vi "Test Snake Created Outside World.vi"(8 "error in (no error)":errorcluster, 11 "Test Case In":refnum<class "World Test.lvclass">) -> (0 "error out":errorcluster, 3 "Test Case Out":refnum<class "World Test.lvclass">)   [LabVIEW 2020, in "World Test.lvclass"]
uses:
  World Test.lvclass
  World Test.lvclass/World Test.ctl
  source/World/World.lvclass
  source/Particle/Position.ctl
  source/Particle.lvclass
  source/Snake/Snake.lvclass
  <vilib>/Astemes/LUnit/Test Case.lvclass
  C:/Program Files (x86)/National Instruments/LabVIEW 2020/vi.lib/Astemes/LUnit/Test Case.lvclass
  C:/git/astemes-snake-game/tests/World Test/World Test.lvclass
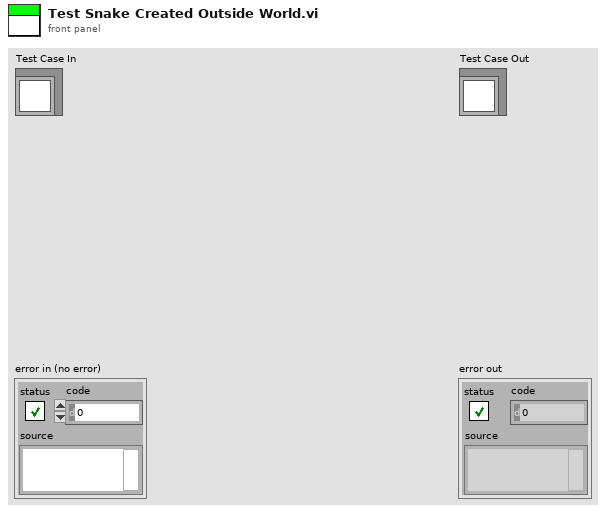
[diagram p1: front panel]
types:
  T1 = typedef "Particle.lvclass/Position.ctl" = cluster{"X":i32, "Y":i32}
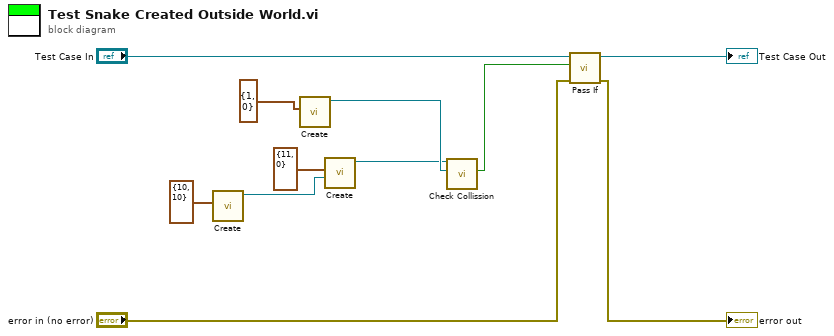
[diagram p0: block diagram]
diagram:
  n1 = call "Create.vi"("Size"=T1 {"X"=10, "Y"=10}) -> ("World out"=w6:refnum<class "World.lvclass">)  [unwired: 10 in]
  n2 = call "Create.vi"("Position"=T1 {"X"=1, "Y"=0}) -> ("Particle out"=w3:refnum<class "Particle.lvclass">)  [unwired: 10 in]
  n3 = call "Create.vi"("World.lvclass"=w6, "Position"=T1 {"X"=11, "Y"=0}) -> ("Snake out"=w1:refnum<class "Snake.lvclass">)  [unwired: 9 in]
  n4 = call "Check Collission.vi"("Particle"=w3, "Snake in"=w1) -> ("Collided?"=w2:bool)  [unwired: 8 in, 1 out]
  n5 = call <vilib>:"Pass If.vi"("error in (no error)"="error in (no error)", "Pass?"=w2, "LUnit Test Case In"="Test Case In") -> ("error out"=→"error out":errorcluster, "LUnit Test Case Out"=→"Test Case Out":refnum<class "World Test.lvclass">)  [unwired: 7 in]
